vi "ConvertMessage.vi"(6 "MessageObjectType":T4, 9 "ServicePrefix":string, 10 "ServiceName":string, 11 "MessageDef in":T1) -> (2 "Message":T3, 3 "MessageDef out":T1)   [LabVIEW 2017, in "MessageGen.lvlib"]
uses:
  <vilib>/addons/InsightCM/MessageBus/CodeGen/MessageGen.lvlib
  <vilib>/addons/InsightCM/MessageBus/CodeGen/controls/MessageDef.ctl
  <vilib>/addons/InsightCM/MessageBus/CodeGen/controls/ParameterDef.ctl
  <vilib>/addons/InsightCM/MessageBus/CodeGen/controls/MessageType.ctl
  <vilib>/addons/InsightCM/MessageBus/CodeGen/controls/MessageData.ctl
  <vilib>/addons/InsightCM/MessageBus/CodeGen/controls/Parameter.ctl
  <vilib>/addons/InsightCM/MessageBus/CodeGen/controls/ParameterType.ctl
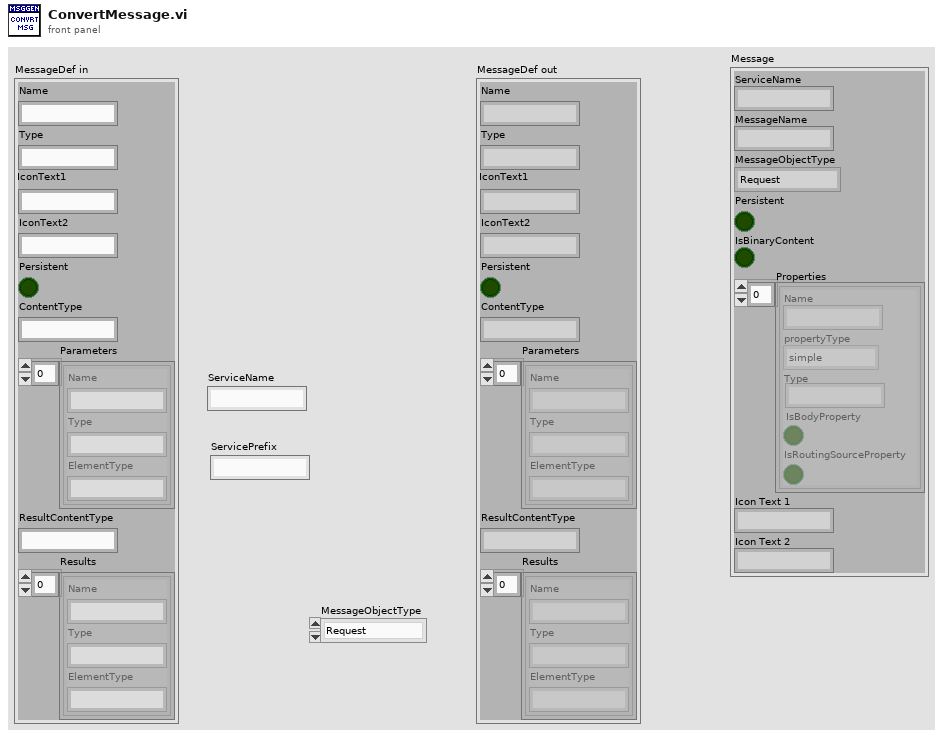
[diagram p1: front panel]
types:
  T1 = typedef "MessageGen.lvlib/MessageDef.ctl" = cluster{"Name":string, "Type":string, "IconText1":string, "IconText2":string, "Persistent":bool, "ContentType":string, "Parameters":T2[], "ResultContentType":string, "Results":T2[]}
  T2 = typedef "MessageGen.lvlib/ParameterDef.ctl" = cluster{"Name":string, "Type":string, "ElementType":string}
  T3 = typedef "MessageGen.lvlib/MessageData.ctl" = cluster{"ServiceName":string, "MessageName":string, "MessageObjectType":T4, "Persistent":bool, "IsBinaryContent":bool, "Properties":T5[], "Icon Text 1":string, "Icon Text 2":string}
  T4 = typedef "MessageGen.lvlib/MessageType.ctl" = enum16{"Request", "Response", "Broadcast", "RoutedMessage"}
  T5 = typedef "MessageGen.lvlib/Parameter.ctl" = cluster{"Name":string, "propertyType":T6, "Type":string, "IsBodyProperty":bool, "IsRoutingSourceProperty":bool}
  T6 = typedef "MessageGen.lvlib/ParameterType.ctl" = enum16{"simple", "bytearray", "dateTime", "list", "map", "object"}
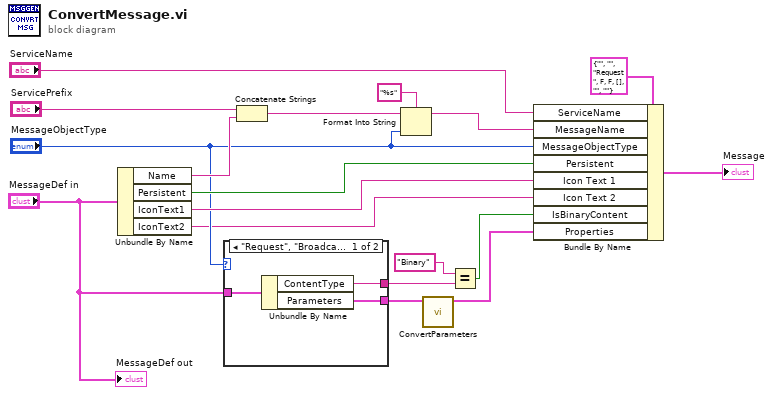
[diagram p0: block diagram]
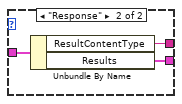
[diagram p2: hidden frame]
diagram:
  n1 = Unbundle By Name("MessageDef in") -> ("Name"=w16:string, "Persistent"=w14:bool, "IconText1"=w13:string, "IconText2"=w1:string)
  n2 = case shown="\"Request\", \"Broadcast\", \"RoutedMessage\"" "MessageObjectType" {
    tunnel: [w20 w23] -> w6
    tunnel: [w19 w22] -> w5
    tunnel: "MessageDef in" -> [w21 w24]
    frame "Request", "Broadcast", "RoutedMessage" {
      n3 = Unbundle By Name(w21) -> ("ContentType"=w20:string, "Parameters"=w19:T2[])
    }
    frame "Response" {
      n4 = Unbundle By Name(w24) -> ("ResultContentType"=w23:string, "Results"=w22:T2[])
    }
  }
  n5 = Concatenate Strings("ServicePrefix", w16) -> (w15:string)
  n6 = Format Into String(format string="%s", initial string=w15, "MessageObjectType") -> (resulting string=w9:string)  [unwired: 1 in, 1 out]
  n7 = call <vilib>:"ConvertParameters.vi"("ParameterDefs"=w5) -> ("Parameters"=w7:T5[])  [unwired: 10 in]
  n8 = Equal?(x="Binary", y=w6) -> (x = y?=w2:bool)
  n9 = Bundle By Name(cluster=T3 {"ServiceName"="", "MessageName"="", "MessageObjectType"=enum."Request", "Persistent"=FALSE, "IsBinaryContent"=FALSE, "Properties"=[], "Icon Text 1"="", "Icon Text 2"=""} ("Message"), "ServiceName"="ServiceName", "MessageName"=w9, "MessageObjectType"="MessageObjectType", "Persistent"=w14, "Icon Text 1"=w13, "Icon Text 2"=w1, "IsBinaryContent"=w2, "Properties"=w7) -> (→"Message":T3)
  "MessageDef out" <- "MessageDef in"
